vi "탭웹브라우저(0).vi"() -> ()   [LabVIEW 2014]
panel:
  out "2":i32
  out "1":i32
  in  "Refresh":u32=2000
  in  "정지":bool
  in  "탭 컨트롤":enum32{"페이지 1", "페이지 2"}(tab)
  in  "WebBrowser":refnum<k7>(container) caption="웹 브라우저"
  in  "WebBrowser 2":refnum<k7>(container) caption="웹 브라우저"
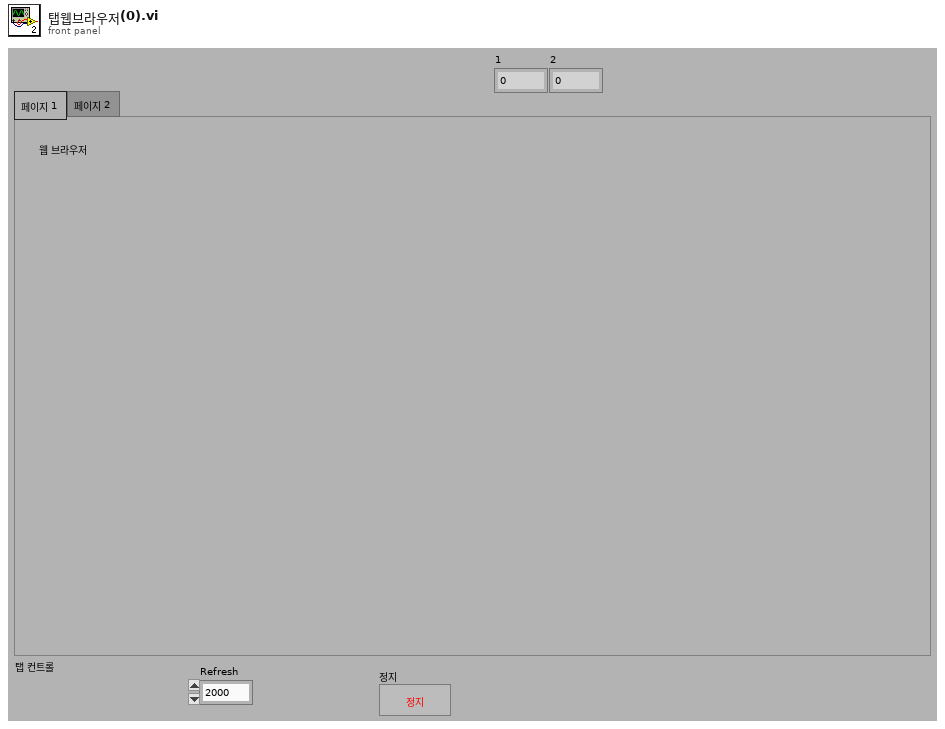
[diagram p1: front panel]
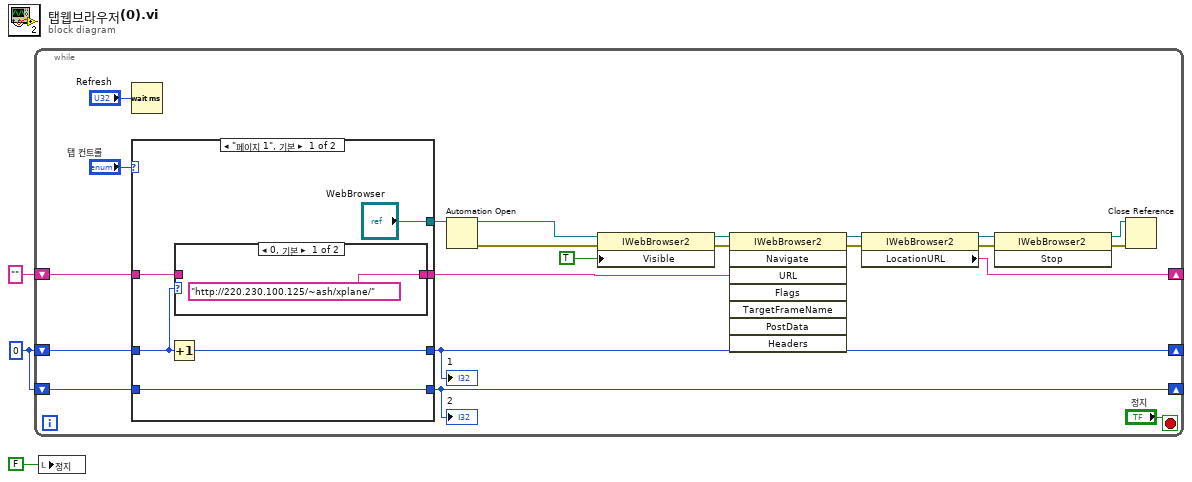
[diagram p0: block diagram]
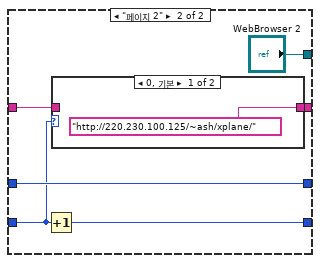
[diagram p3: hidden frame]
diagram:
  w2 = 0
  n1 = while {
    shift-right: [w15] -> _
    shift-left: "" ("LocationURL") -> [w14]
    shift-right: [w10] -> _
    shift-left: w2 -> [w11]
    shift-right: [w12] -> _
    shift-left: w2 -> [w13]
    stop <- "정지" stop-if-true
    n2 = Wait (ms)(milliseconds to wait="Refresh") -> ()  [unwired: 1 out]
    n3 = case shown="\"페이지 1\", 기본" "탭 컨트롤" {
      tunnel: ["WebBrowser" "WebBrowser 2"] -> w20
      tunnel: [w30 w38] -> w22
      tunnel: w14 -> [w29 w36]
      tunnel: w13 -> [w26 w37]
      tunnel: [w28 w37] -> w12
      tunnel: w11 -> [w27 w34]
      tunnel: [w27 w35] -> w10
      frame "페이지 1", Default {
        n4 = Increment(x=w26) -> (x+1=w28:i32)
        n5 = case shown="0, 기본" w26 {
          tunnel: ["http://220.230.100.125/~ash/xplane/" w33] -> w30
          tunnel: w29 -> [_ w33]
          frame 0, Default {
          }
          frame 1.. {
          }
        }
      }
      frame "페이지 2" {
        n6 = Increment(x=w34) -> (x+1=w35:i32)
        n7 = case shown="0, 기본" w34 {
          tunnel: ["http://220.230.100.125/~ash/xplane/" w41] -> w38
          tunnel: w36 -> [_ w41]
          frame 0, Default {
          }
          frame 1.. {
          }
        }
      }
    }
    "1" <- w12
    "2" <- w10
    n8 = Automation Open(Automation Refnum=w20) -> (Automation Refnum=w19:refnum<k7>, error out=w18:errorcluster)  [unwired: 1 in, 2 out]
    n9 = property class="IWebBrowser2"(reference=w19, error in=w18, "Visible"=TRUE) -> (reference out=w23:refnum<k7>, error out=w24:errorcluster)
    n10 = invoke class="IWebBrowser2" method="Navigate"(reference=w23, error in=w24, "URL"=w22) -> (reference out=w9:refnum<k7>, error out=w8:errorcluster)  [unwired: 5 in, 6 out]
    n11 = property class="IWebBrowser2"(reference=w9, error in=w8) -> (reference out=w7:refnum<k7>, error out=w6:errorcluster, "LocationURL"=w15:string)
    n12 = invoke class="IWebBrowser2" method="Stop"(reference=w7, error in=w6) -> (reference out=w4:refnum<k7>, error out=w5:errorcluster)  [unwired: 1 in, 1 out]
    n13 = Close Reference(reference=w4, error in (no error)=w5) -> ()  [unwired: 1 out]
  }
  n14 = local write "정지"(FALSE ("정지")) -> ()
